vi "Configure Measurement (AM Noise).vi"(0 "VISA resource name":refnum<visa-resource-name>, 1 "Spurious Mode (0: Normalized)":u16(ring) items=["Normalized (dBc/Hz)", "Power (dBc)", "Omit"], 7 "Correlation (1)":i32=1, 11 "error in (no error)":errorcluster, 12 "Minimum Spur Level (-500 dBc)":dbl=-500.0 format="%^#_9g") -> (4 "VISA resource name out":refnum<visa-resource-name>, 15 "error out":errorcluster)   [LabVIEW 2011, in "Agilent E5052X.lvlib"]
doc: "Configures the instrument to take AM Noise measurements.\n\n<b>Note: </b>\n\n1) AM Noise Measurement is not available for the E5052A signal source analyzer.\n\n2) \"Configure Measurement Characteristics(AM Noise)\" VI must be called before calling this VI."
uses:
  Agilent E5052X.lvlib
panel:
  # "Spurious Settings"
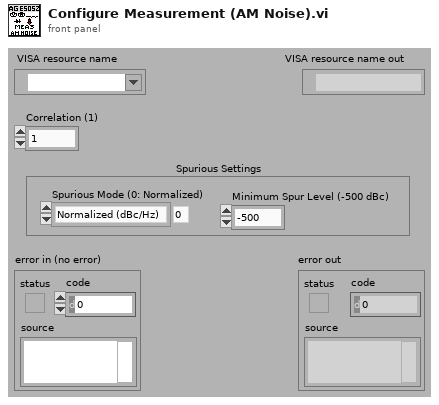
[diagram p1: front panel]
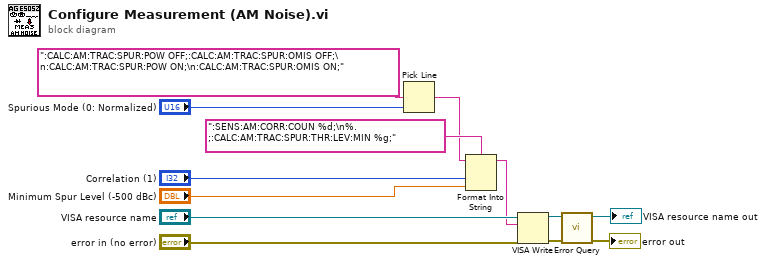
[diagram p0: block diagram]
diagram:
  n1 = Pick Line(multi-line string=":CALC:AM:TRAC:SPUR:POW OFF;:CALC:AM:TRAC:SPUR:OMIS OFF;\n:CALC:AM:TRAC:SPUR:POW ON;\n:CALC:AM:TRAC:SPUR:OMIS ON;", line index="Spurious Mode (0: Normalized)") -> (output string=w2:string)  [unwired: 1 in]
  n2 = Format Into String(format string=":SENS:AM:CORR:COUN %d;\n%.;:CALC:AM:TRAC:SPUR:THR:LEV:MIN %g;", initial string=w2, "Correlation (1)", "Minimum Spur Level (-500 dBc)") -> (resulting string=w1:string)  [unwired: 1 in, 1 out]
  n3 = VISA Write(VISA resource name="VISA resource name", write buffer=w1, error in (no error)="error in (no error)") -> (VISA resource name out=w8:refnum<visa-resource-name>, error out=w7:errorcluster)  [unwired: 1 out]
  n4 = call "Error Query.vi"("error in (no error)"=w7, "VISA resource name"=w8) -> ("error out"=→"error out":errorcluster, "VISA resource name out"=→"VISA resource name out":refnum<visa-resource-name>)  [unwired: 6 in, 2 out]
